vi "ABRE ARCHIVO.vi"(0 "File Path Control":path, 11 "error in (no error)":errorcluster) -> (3 "Número de datos":i32, 4 "EJE X":dbl[](array[numeric]), 6 "EJE Y":dbl[](array[numeric]), 8 "Ángulo máximo":dbl, 10 "Ángulo mínimo":dbl, 15 "error out":errorcluster)   [LabVIEW 2025]
uses:
  <vilib>/Utility/file.llb/Read Delimited Spreadsheet (DBL).vi
panel:
  out "EJE X y Y":dbl[][](array[numeric])
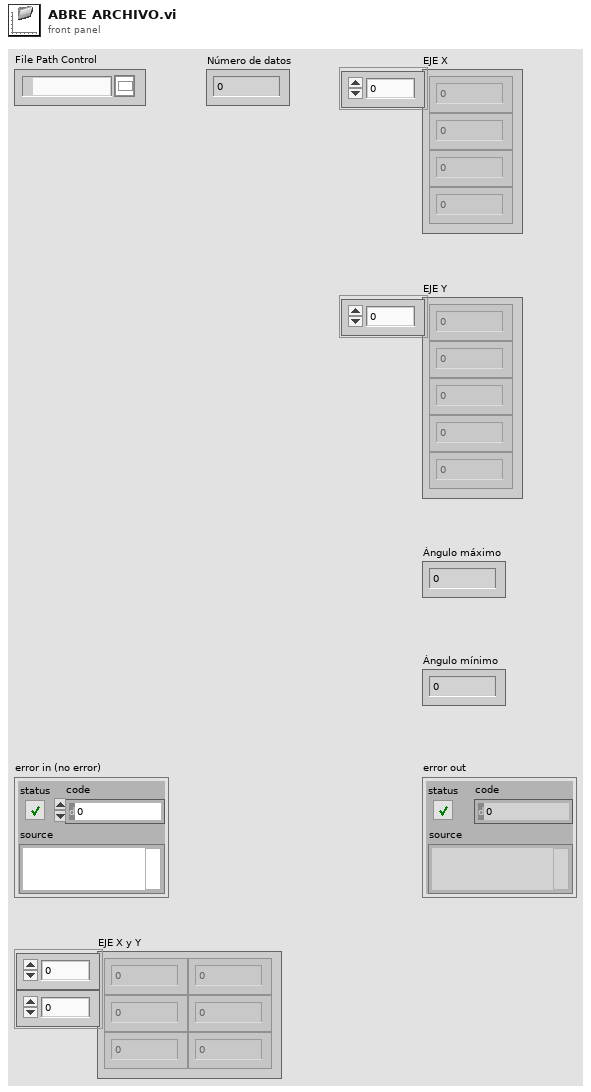
[diagram p1: front panel]
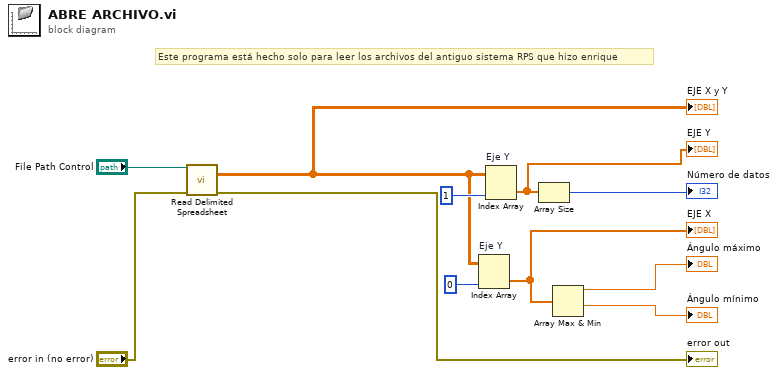
[diagram p0: block diagram]
diagram:
  # "Este programa está hecho solo para leer los archivos del antiguo sistema RPS que hizo enrique"
  n1 = call-poly <vilib>:"Read Delimited Spreadsheet.vi"("file path (dialog if empty)"="File Path Control", "error in (no error)"="error in (no error)") -> ("all rows"=w5:dbl[][], "error out"=→"error out":errorcluster)  [unwired: 8 in, 4 out]
  "EJE X y Y" <- w5
  n2 = Index Array "Eje Y"(array=w5, index (col)=0 ("length")) -> (element=w4:dbl[])  [unwired: 1 in]
  "EJE X" <- w4
  n3 = Index Array "Eje Y"(array=w5, index (col)=1 ("index")) -> (element=w6:dbl[])  [unwired: 1 in]
  "EJE Y" <- w6
  n4 = Array Size(array=w6) -> (size(s)=→"Número de datos":i32)
  n5 = Array Max & Min(array=w4) -> (max value=→"Ángulo máximo":dbl, min value=→"Ángulo mínimo":dbl)  [unwired: 2 out]
